vi "Intake Controller.vi"(8 "error in":errorcluster) -> ()   [LabVIEW 2017]
doc: "This VI executes continuously carrying out the current operation and responding to updates or new operations. It will often contain the timing or control code that is difficult to place directly in TeleOp. This VI generally opens all sensors and motors and isolates the rest of the robot code from knowing how the operations are carried out."
uses:
  <vilib>/Rock Robotics/WPI/Framework/Completion Status.ctl
  Intake Setpoints.ctl
  Intake Operations.ctl
  <vilib>/Rock Robotics/WPI/SafetyOutput/WPI_SafetyOutputConfigMenu.ctl
  <vilib>/Rock Robotics/Network Tables/NT Write Boolean.vi
panel:
  in  "haveCube (sensor)":bool
  in  "Interactive Values":T1
  out "Current\nCmd":string
  in  "Buttons":cluster{"Execute Cmd":bool, "Abort Cmd":bool}
  out "Command Timing":cluster{"Start Time (ms)":u32, "Iterations":i32}
  out "Status":T3
  # "Tip: It may be helpful to observe inputs and sensor values.\nYou may also want to display tuning or debugging controls."
  # "Interactive Command: You may fill in the settings for a command\nand schedule it with the Execute button. You can observe and abort\nany command while fine tuning the code for the controller."
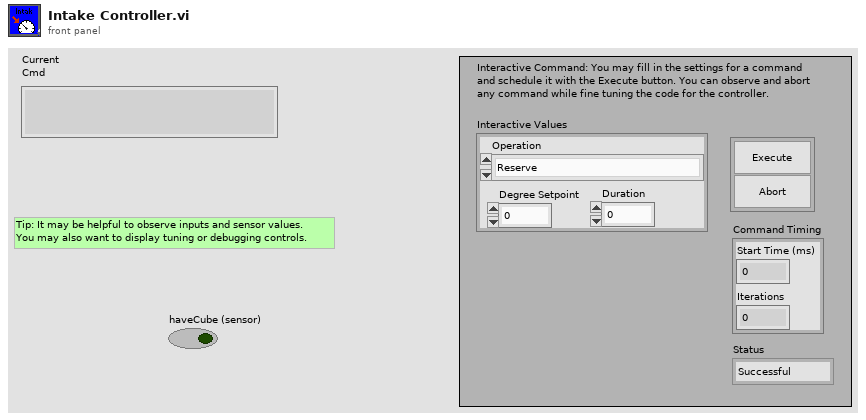
[diagram p1: front panel]
types:
  T1 = typedef "Intake Setpoints.ctl" = cluster{"Operation":T2, "Degree Setpoint":dbl, "Duration":dbl}
  T2 = typedef "Intake Operations.ctl" = enum16{"Reserve", "Read Current", "setSetpoint", "feed", "spit"}
  T3 = typedef "Completion Status.ctl" = enum16{"Successful", "Aborted", "Incomplete"}
  T4 = typedef "WPI_SafetyOutputConfigMenu.ctl" = enum16{"Enable", "Disable"}
  T5 = typedef "WPI_MotorControlDeviceRef.ctl" = cluster{"DeviceStatus":errorcluster, "Type":T6, "PWM":cluster{"PWM Channel":T7, "DeadBand":T8}, "CAN":cluster{"Device Number":u8, "SetOutput VI Ref":variant, "GetOutput VI Ref":variant, "Enable VI Ref":variant, "Disable VI Ref":variant, "Data":variant}, "Invert":bool, "DIO PWM":cluster{"PWM \"Enable\" Channel":T7, "DIOChannel":T9, "PWM Rate":dbl}}
  T6 = typedef "WPI_MotorControlType.ctl" = enum16{"PWM", "CAN", "DIO PWM"}
  T7 = typedef "FPGA_DIOPWMChannel.ctl" = enum8{"PWM 0", "PWM 1", "PWM 2", "PWM 3", "PWM 4", "PWM 5", "PWM 6", "PWM 7", "PWM 8", "PWM 9", "PWM MXP 0", "PWM MXP 1", "PWM MXP 2", "PWM MXP 3", "PWM MXP 4", "PWM MXP 5", "PWM MXP 6", "PWM MXP 7", "PWM MXP 8", "PWM MXP 9", "Invalid"}
  T8 = typedef "WPI_PWMDeadband.ctl" = cluster{"Name":string, "maxPositivePwm":i32, "minPositivePwm":i32, "centerPwm":i32, "maxNegativePwm":i32, "minNegativePwm":i32, "angularRange":u16}
  T9 = typedef "FPGA_DIOChannel.ctl" = enum8{"DIO 0", "DIO 1", "DIO 2", "DIO 3", "DIO 4", "DIO 5", "DIO 6", "DIO 7", "DIO 8", "DIO 9", "DIO MXP 0", "DIO MXP 1", "DIO MXP 2", "DIO MXP 3", "DIO MXP 4", "DIO MXP 5", "DIO MXP 6", "DIO MXP 7", "DIO MXP 8", "DIO MXP 9", "DIO MXP 10", "DIO MXP 11", "DIO MXP 12", "DIO MXP 13", "DIO MXP 14", "DIO MXP 15", "SPI Port CS1", "SPI Port CS2", "SPI Port CS3", "SPI Port MISO", "SPI Port MOSI", "Invalid"}
  T10 = typedef "WPI_PotentiometerDevRef.ctl" = cluster{"DevStatus":errorcluster, "Analog Channel":T11, "Invert Output":bool}
  T11 = typedef "FPGA_AIChannel.ctl" = enum8{"AI 0", "AI 1", "AI 2", "AI 3", "AI MXP 0", "AI MXP 1", "AI MXP 2", "AI MXP 3", "Invalid"}
  T12 = typedef "Command Status Info.ctl" = cluster{"Name":string, "Status":T3, "notifier out":T13}
  T13 = typedef "Completion Notifier.ctl" = refnum<notifier>
  T14 = cluster{"Current Command":T1, "Command Timing":cluster{"Start Time (ms)":u32, "Iterations":i32}, "Command Arguments":cluster{"Command Info":T12, "Description":string, "Default Command":T1, "queue out":refnum<queue>, "Subsystem Name":string}}
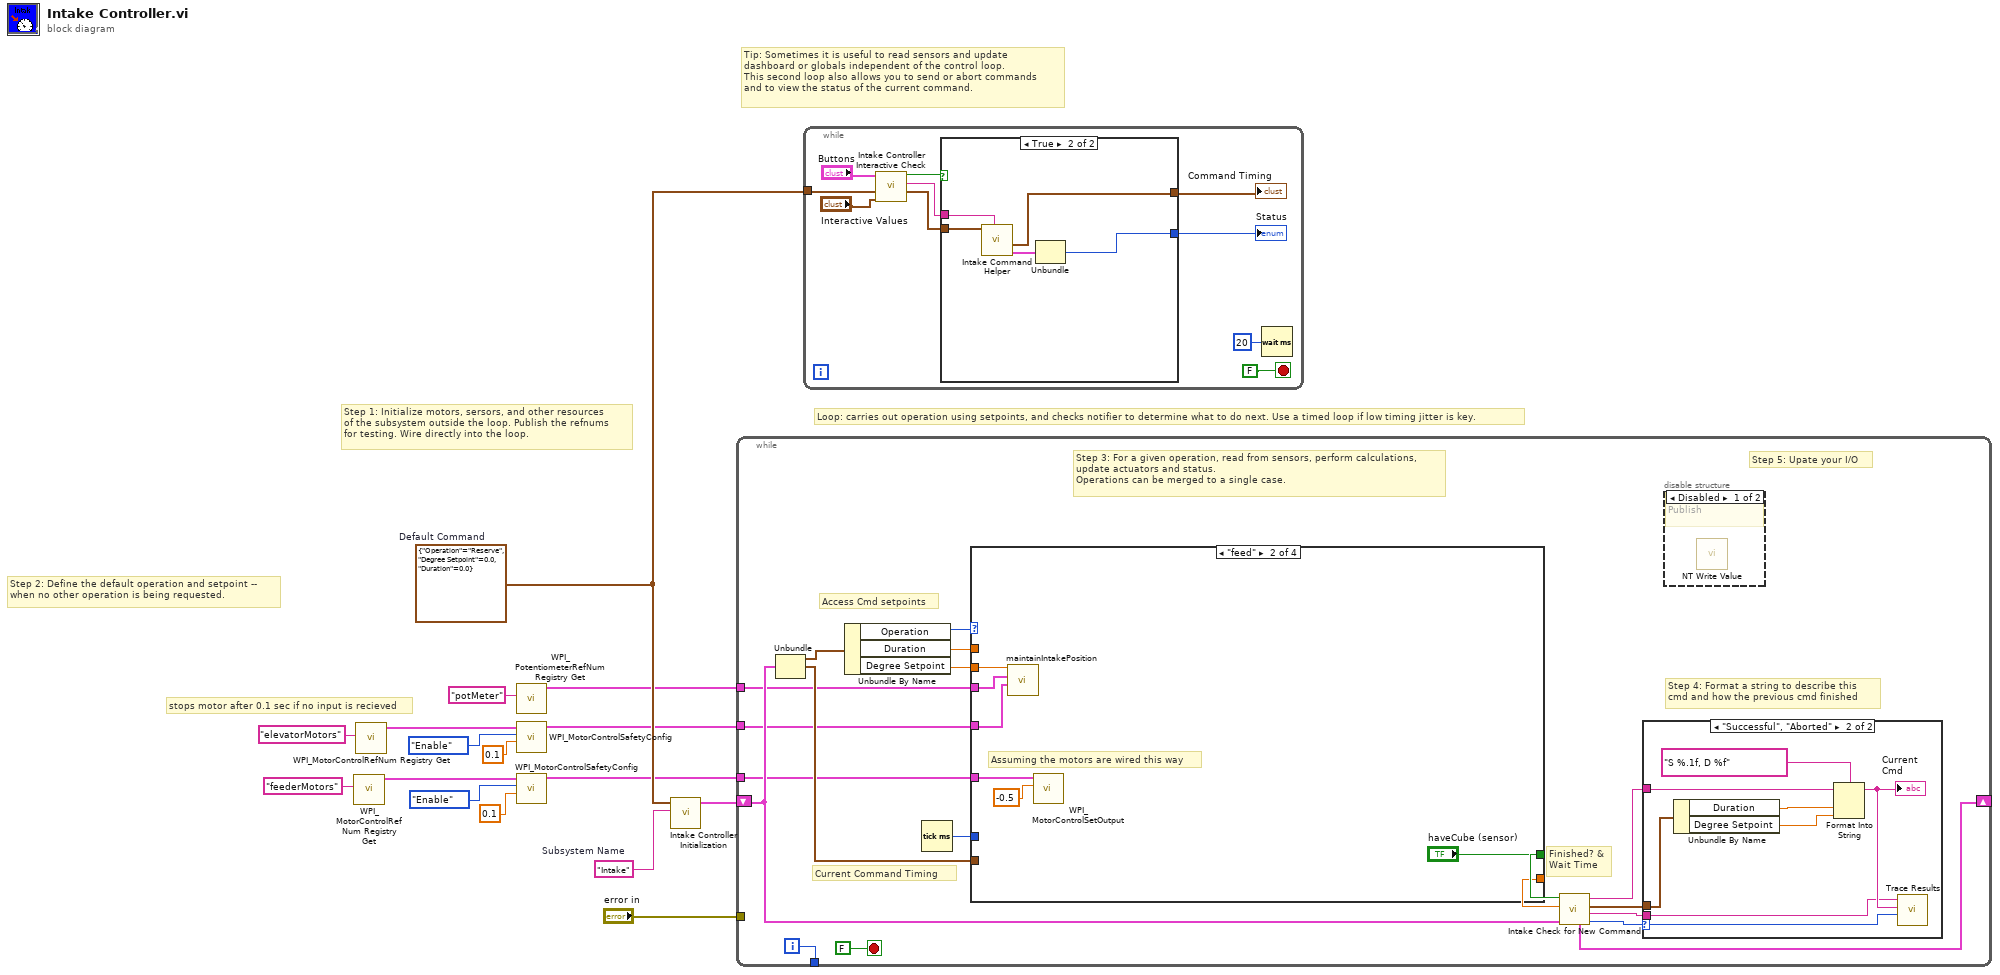
[diagram p0: block diagram]
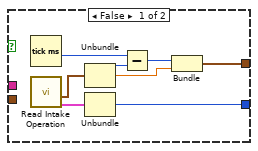
[diagram p2: hidden frame]
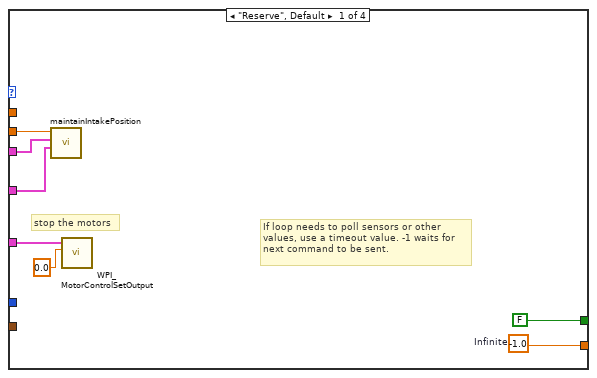
[diagram p5: hidden frame]
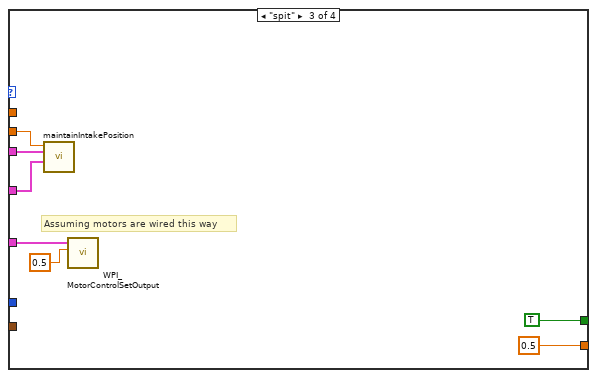
[diagram p6: hidden frame]
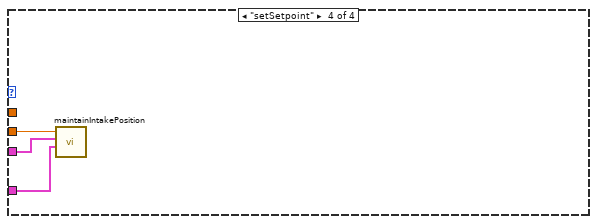
[diagram p7: hidden frame]
diagram:
  w13 = T1 {"Operation"=enum."Reserve", "Degree Setpoint"=0.0, "Duration"=0.0}  # Default Command
  w14 = "Intake"  # Subsystem Name
  # "stops motor after 0.1 sec if no input is recieved"
  # "Tip: Sometimes it is useful to read sensors and update\ndashboard or globals independent of the control loop.\nThis second loop also allows you to send or abort commands\nand to view the status of the current command."
  # "Step 2: Define the default operation and setpoint --\nwhen no other operation is being requested."
  # "Step 1: Initialize motors, sersors, and other resources\nof the subsystem outside the loop. Publish the refnums\nfor testing. Wire directly into the loop."
  # "Loop: carries out operation using setpoints, and checks notifier to determine what to do next. Use a timed loop if low timing jitter is key."
  n1 = call <vilib>:"WPI_MotorControlRefNum Registry Get.vi"("refnum name"="feederMotors") -> ("MotorControlDevRef"=w9:T5)  [unwired: 9 in, 1 out]
  n2 = call <vilib>:"WPI_MotorControlRefNum Registry Get.vi"("refnum name"="elevatorMotors") -> ("MotorControlDevRef"=w12:T5)  [unwired: 9 in, 1 out]
  n3 = call <vilib>:"WPI_PotentiometerRefNum Registry Get.vi"("refnum name"="potMeter") -> ("PotDevRef"=w5:T10)  [unwired: 9 in, 1 out]
  n4 = call <vilib>:"WPI_MotorControlSafetyConfig.vi"("timeout (s)"=0.1, "mode"=WPI_SafetyOutputConfigMenu."Enable", "MotorControlDevRef"=w12) -> ("MotorControlDevRef"=w4:T5)  [unwired: 7 in, 1 out]
  n5 = call <vilib>:"WPI_MotorControlSafetyConfig.vi"("timeout (s)"=0.1, "mode"=WPI_SafetyOutputConfigMenu."Enable", "MotorControlDevRef"=w9) -> ("MotorControlDevRef"=w1:T5)  [unwired: 7 in, 1 out]
  n6 = call "Intake Controller Initialization.vi"("Subsystem Name"=w14, "Default Command"=w13) -> ("Current Command"=w15:T14)  [unwired: 9 in]
  n7 = while {
    shift-right: [w27] -> _
    shift-left: w15 -> [w20]
    tunnel: [w34] -> _
    tunnel: "error in" -> [_]
    tunnel: w5 -> [w19]
    tunnel: w4 -> [w18]
    tunnel: w1 -> [w17]
    i -> [w34]
    stop <- FALSE stop-if-true
    # "Step 5: Upate your I/O"
    # "Step 4: Format a string to describe this\ncmd and how the previous cmd finished"
    # "Current Command Timing"
    # "Access Cmd setpoints"
    # "Finished? &\nWait Time"
    # "Step 3: For a given operation, read from sensors, perform calculations,\nupdate actuators and status.\nOperations can be merged to a single case."
    n8 = Unbundle(w20) -> ("Current Command"=w33:T1, "Command Timing"=w29:cluster{"Start Time (ms)":u32, "Iterations":i32})  [unwired: 1 out]
    n9 = Unbundle By Name(w33) -> ("Operation"=w32:T2, "Duration"=w31:dbl, "Degree Setpoint"=w28:dbl)
    n10 = Tick Count (ms)() -> (millisecond timer value=w30:u32)
    n11 = case shown="\"feed\"" w32 {
      tunnel: [w50 _ 0.5 ("Infinite") _] -> w25
      tunnel: [FALSE ("ignore previous (F)") "haveCube (sensor)" TRUE ("ignore previous (F)") _] -> w26
      tunnel: w29 -> [_ _ _ _]
      tunnel: w31 -> [_ _ _ _]
      tunnel: w30 -> [_ _ _ _]
      tunnel: w28 -> [w48 w56 w63 w66]
      tunnel: w19 -> [w47 w55 w62 w65]
      tunnel: w18 -> [w46 w54 w61 w64]
      tunnel: w17 -> [w44 w52 w58 _]
      frame "Reserve", Default {
        w50 = -1.0  # Infinite
        # "stop the motors"
        # "If loop needs to poll sensors or other\nvalues, use a timeout value. -1 waits for\nnext command to be sent."
        n12 = call "maintainIntakePosition.vi"("MotorControlDevRef"=w46, "PotDevRef"=w47, "Degree Setpoint"=w48) -> ()  [unwired: 9 in]
        n13 = call <vilib>:"WPI_MotorControlSetOutput.vi"("Output"=0.0, "MotorControlDevRef"=w44) -> ()  [unwired: 7 in, 3 out]
      }
      frame "feed" {
        # "Assuming the motors are wired this way"
        n14 = call "maintainIntakePosition.vi"("MotorControlDevRef"=w54, "PotDevRef"=w55, "Degree Setpoint"=w56) -> ()  [unwired: 9 in]
        n15 = call <vilib>:"WPI_MotorControlSetOutput.vi"("Output"=-0.5, "MotorControlDevRef"=w52) -> ()  [unwired: 7 in, 3 out]
      }
      frame "spit" {
        # "Assuming motors are wired this way"
        n16 = call "maintainIntakePosition.vi"("MotorControlDevRef"=w61, "PotDevRef"=w62, "Degree Setpoint"=w63) -> ()  [unwired: 9 in]
        n17 = call <vilib>:"WPI_MotorControlSetOutput.vi"("Output"=0.5, "MotorControlDevRef"=w58) -> ()  [unwired: 7 in, 3 out]
      }
      frame "setSetpoint" {
        n18 = call "maintainIntakePosition.vi"("MotorControlDevRef"=w64, "PotDevRef"=w65, "Degree Setpoint"=w66) -> ()  [unwired: 9 in]
      }
    }
    n19 = call "Intake Check for New Command.vi"("Current Command"=w20, "Wait time (ms)"=w25, "Finished?"=w26) -> ("Completion"=w21:T3, "Subsystem Name"=w22:string, "Current Command"=w23:T1, "Initial Trace String"=w24:string, "NextCommand"=w27:T14)  [unwired: 4 in]
    n20 = case shown="\"Successful\", \"Aborted\"" w21 {
      selector: w21 -> [_ w43]
      tunnel: w24 -> [_ w39]
      tunnel: w23 -> [_ w40]
      tunnel: w22 -> [_ w36]
      frame "Incomplete", Default {
        # "Continuing current command"
      }
      frame "Successful", "Aborted" {
        # "Report and setup for next command"
        n21 = Unbundle By Name(w40) -> ("Duration"=w42:dbl, "Degree Setpoint"=w37:dbl)
        n22 = Format Into String(format string="S %.1f, D %f", initial string=w39, w42, w37) -> (resulting string=w38:string)  [unwired: 1 in, 1 out]
        "Current\nCmd" <- w38
        n23 = call <vilib>:"Trace Results.vi"("Status of previous command"=w43, "Description"=w38, "Subsystem"=w36) -> ()  [unwired: 9 in]
      }
    }
    n24 = disable-structure shown="Disabled" {
      frame Disabled {
        # "Publish"
        n25 = call-poly <vilib>:"NT Write Value.vi"() -> ()  [unwired: 11 in, 1 out]
      }
      frame Enabled {
      }
    }
  }
  n26 = while {
    tunnel: w13 -> [w73]
    stop <- FALSE stop-if-true
    n27 = call "Intake Controller Interactive Check.vi"("Interactive Command in"="Interactive Values", "Default Command"=w73, "Buttons"="Buttons") -> ("Interactive Command out"=w70:T1, "Trace String"=w71:string, "Schedule"=w72:bool)  [unwired: 6 in]
    n28 = case shown="True" w72 {
      tunnel: [w84 w89] -> w69
      tunnel: w70 -> [_ w87]
      tunnel: [w80 w85] -> w68
      tunnel: w71 -> [_ w88]
      frame False {
        n29 = Tick Count (ms)() -> (millisecond timer value=w79:u32)
        n30 = call "Read Intake Operation.vi"() -> ("Command Info"=w77:T12, "SubSystem Data"=w78:T1)  [unwired: 9 in, 1 out]
        n31 = Unbundle(w78) -> ("Operation"=w83:T2, "Degree Setpoint"=w81:dbl)  [unwired: 1 out]
        n32 = Unbundle(w77) -> ("Status"=w84:T3)  [unwired: 2 out]
        n33 = Subtract(x=w79, y=w83) -> (x-y=w82:u32)
        n34 = Bundle(w82, "Degree Setpoint"=w81) -> (w80:cluster{u32, "Degree Setpoint":dbl})  [unwired: 1 in]
      }
      frame True {
        n35 = call "Intake Command Helper.vi"("Description"=w88, "SubSystem Data"=w87) -> ("Command Info Out"=w86:T12, "Command Timing"=w85:cluster{"Start Time (ms)":u32, "Iterations":i32})  [unwired: 7 in, 1 out]
        n36 = Unbundle(w86) -> ("Status"=w89:T3)  [unwired: 2 out]
      }
    }
    "Status" <- w69
    "Command Timing" <- w68
    n37 = Wait (ms)(milliseconds to wait=u32 20) -> ()  [unwired: 1 out]
  }
